vi "Vision Auto Move Straight.vi"(6 "Target Angle":dbl, 7 "Target Distance":dbl=15.0 format="%#_13g", 8 "Error In":errorcluster, 11 "Refnum's In":T1) -> (0 "Error Out":errorcluster, 3 "Refnum's Out":T1)   [LabVIEW 2018]
uses:
  <vilib>/Rock Robotics/WPI/ThirdParty/Phoenix-LabVIEW/Controls/CTRE_Phoenix_Params.ctl
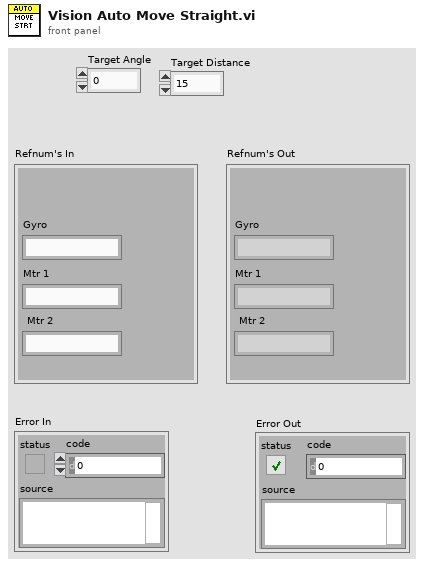
[diagram p1: front panel]
types:
  T1 = cluster{"Gyro":string, "Mtr 1":string, "Mtr 2":string}
  T2 = typedef "WPI_MotorControlDeviceRef.ctl" = cluster{"DeviceStatus":errorcluster, "Type":T3, "PWM":cluster{"PWM Channel":T4, "DeadBand":T5}, "CAN":cluster{"Device Number":u8, "SetOutput VI Ref":variant, "GetOutput VI Ref":variant, "Enable VI Ref":variant, "Disable VI Ref":variant, "Data":variant}, "Invert":bool, "DIO PWM":cluster{"PWM \"Enable\" Channel":T4, "DIOChannel":T6, "PWM Rate":dbl}}
  T3 = typedef "WPI_MotorControlType.ctl" = enum16{"PWM", "CAN", "DIO PWM"}
  T4 = typedef "FPGA_DIOPWMChannel.ctl" = enum8{"PWM 0", "PWM 1", "PWM 2", "PWM 3", "PWM 4", "PWM 5", "PWM 6", "PWM 7", "PWM 8", "PWM 9", "PWM MXP 0", "PWM MXP 1", "PWM MXP 2", "PWM MXP 3", "PWM MXP 4", "PWM MXP 5", "PWM MXP 6", "PWM MXP 7", "PWM MXP 8", "PWM MXP 9", "Invalid"}
  T5 = typedef "WPI_PWMDeadband.ctl" = cluster{"Name":string, "maxPositivePwm":i32, "minPositivePwm":i32, "centerPwm":i32, "maxNegativePwm":i32, "minNegativePwm":i32, "angularRange":u16}
  T6 = typedef "FPGA_DIOChannel.ctl" = enum8{"DIO 0", "DIO 1", "DIO 2", "DIO 3", "DIO 4", "DIO 5", "DIO 6", "DIO 7", "DIO 8", "DIO 9", "DIO MXP 0", "DIO MXP 1", "DIO MXP 2", "DIO MXP 3", "DIO MXP 4", "DIO MXP 5", "DIO MXP 6", "DIO MXP 7", "DIO MXP 8", "DIO MXP 9", "DIO MXP 10", "DIO MXP 11", "DIO MXP 12", "DIO MXP 13", "DIO MXP 14", "DIO MXP 15", "SPI Port CS1", "SPI Port CS2", "SPI Port CS3", "SPI Port MISO", "SPI Port MOSI", "Invalid"}
  T7 = typedef "WPI_GyroDevRef.ctl" = cluster{"DevStatus":errorcluster, "Analog Channel":T8, "Gain (VoltsPerDegree/Second)":dbl, "Gyro Type":enum16{"Analog", "XRS450"}, "Handle":i32, "SPI Bus":T9, "Device Found":bool, "Sample Rate":dbl, "Calibrate On Open":bool, "Offset":dbl}
  T8 = typedef "FPGA_AIChannel.ctl" = enum8{"AI 0", "AI 1", "AI 2", "AI 3", "AI MXP 0", "AI MXP 1", "AI MXP 2", "AI MXP 3", "Invalid"}
  T9 = typedef "spi_bus.ctl" = enum16{"SPI On-Board, CS0", "SPI On-Board, CS1", "SPI On-Board, CS2", "SPI On-Board, CS3", "SPI MXP", "Invalid"}
  T10 = typedef "CTRE_Phoenix_Params.ctl" = u16
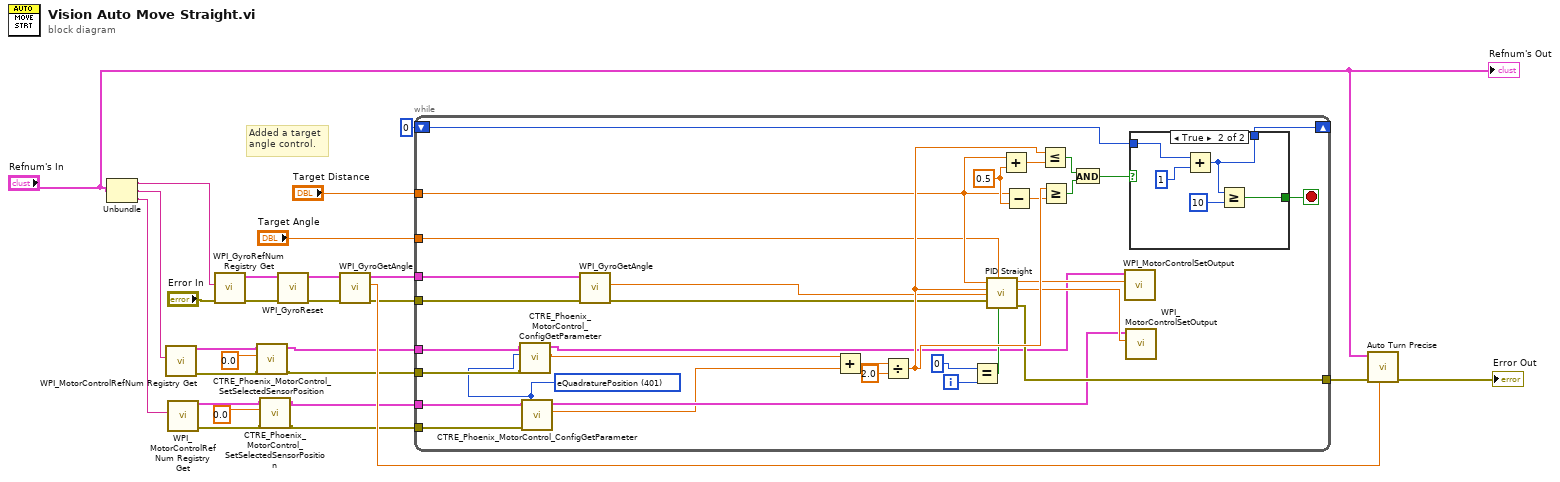
[diagram p0: block diagram]
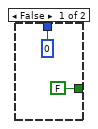
[diagram p2: hidden frame]
diagram:
  # "Added a target\nangle control."
  n1 = Unbundle("Refnum's In") -> ("Gyro"=w13:string, "Mtr 1"=w12:string, "Mtr 2"=w11:string)
  n2 = call <vilib>:"WPI_MotorControlRefNum Registry Get.vi"("refnum name"=w12) -> ("error out"=w4:errorcluster, "MotorControlDevRef"=w5:T2)  [unwired: 9 in]
  n3 = call <vilib>:"WPI_MotorControlRefNum Registry Get.vi"("refnum name"=w11) -> ("error out"=w7:errorcluster, "MotorControlDevRef"=w10:T2)  [unwired: 9 in]
  n4 = call <vilib>:"WPI_GyroRefNum Registry Get.vi"("error in (no error)"="Error In", "refnum name"=w13) -> ("error out"=w18:errorcluster, "GyroDevRef"=w17:T7)  [unwired: 8 in]
  n5 = call <vilib>:"CTRE_Phoenix_MotorControl_SetSelectedSensorPosition.vi"("error in (no error)"=w4, "New Sensor Position"=0.0, "PhoenixMotorControlDevRef"=w5) -> ("error out"=w3:errorcluster, "PhoenixMotorControlDevRef"=w2:T2)  [unwired: 7 in]
  n6 = call <vilib>:"CTRE_Phoenix_MotorControl_SetSelectedSensorPosition.vi"("error in (no error)"=w7, "New Sensor Position"=0.0, "PhoenixMotorControlDevRef"=w10) -> ("error out"=w8:errorcluster, "PhoenixMotorControlDevRef"=w9:T2)  [unwired: 7 in]
  n7 = call <vilib>:"WPI_GyroReset.vi"("error in"=w18, "GyroDevRef"=w17) -> ("error out"=w16:errorcluster, "GyroDevRef"=w15:T7)  [unwired: 8 in]
  n8 = call <vilib>:"WPI_GyroGetAngle.vi"("error in"=w16, "GyroDevRef"=w15) -> ("error out"=w20:errorcluster, "Angle"=w21:dbl, "GyroDevRef"=w19:T7)  [unwired: 5 in, 2 out]
  n9 = while {
    shift-right: [w49] -> _
    shift-left: 0 -> [w48]
    tunnel: "Target Distance" -> [w38]
    tunnel: [w44] -> w26
    tunnel: "Target Angle" -> [w37]
    tunnel: w19 -> [w40]
    tunnel: w20 -> [w39]
    tunnel: w8 -> [w35]
    tunnel: w9 -> [w36]
    tunnel: w3 -> [w32]
    tunnel: w2 -> [w33]
    i -> [w60]
    stop <- w43 stop-if-true
    w28 = T10 401 items=["eOnBoot_BrakeMode"=31, "eQuadFilterEn"=91, "eQuadIdxPolarity"=108, "eClearPositionOnIdx"=100, "eMotionProfileHasUnderrunErr"=119, "eMotionProfileTrajectoryPointDurationMs"=120, "eClearPosOnLimitF"=144, "eClearPosOnLimitR"=145, "eStatusFramePeriod"=300, "eOpenLoopRamp"=301, "eClosedLoopRamp"=302, "eNeutralDeadband"=303, "ePeakPosOutput"=305, "eNominalPosOutput"=306, "ePeakNegOutput"=307, "eNominalNegOutput"=308, "eProfileParamSlot_P"=310, "eProfileParamSlot_I"=311, "eProfileParamSlot_D"=312, "eProfileParamSlot_F"=313, "eProfileParamSlot_IZone"=314, "eProfileParamSlot_AllowableErr"=315, "eProfileParamSlot_MaxIAccum"=316, "eProfileParamSlot_PeakOutput"=317, "eClearPositionOnLimitF"=320, "eClearPositionOnLimitR"=321, "eClearPositionOnQuadIdx"=322, "eSampleVelocityPeriod"=325, "eSampleVelocityWindow"=326, "eFeedbackSensorType"=330, "eSelectedSensorPosition"=331, "eFeedbackNotContinuous"=332, "eRemoteSensorSource"=333, "eRemoteSensorDeviceID"=334, "eSensorTerm"=335, "eRemoteSensorClosedLoopDisableNeutralOnLOS"=336, "ePIDLoopPolarity"=337, "ePIDLoopPeriod"=338, "eSelectedSensorCoefficient"=339, "eForwardSoftLimitThreshold"=340, "eReverseSoftLimitThreshold"=341, "eForwardSoftLimitEnable"=342, "eReverseSoftLimitEnable"=343, "eNominalBatteryVoltage"=350, "eBatterVoltageFilterSize"=351, "eContinuousCurrentLimitAmps"=360, "eContinuousCurrentLimitMs"=361, "ePeakCurrentLimitAmps"=362, "eClosedLoopIAccum"=370, "eCustomParam"=380, "eStickyFaults"=390, "eAnalogPosition"=400, "eQuadraturePosition"=401, "ePulseWidthPosition"=402, "eMotMag_Accel"=410, "eMotMag_VelCruise"=411, "eLimitSwitchSource"=421, "eLimitSwitchNormClosedAndDis"=422, "eLimitSwitchDisabledNeutralOnLOS"=423, "eLimitSwitchRemoteDevID"=424, "eSoftLimitDisabledNeutralOnLOS"=425, "ePulseWidthPeriod_EdgesPerRot"=430, "ePulseWidthPeriod_FilterWindowSz"=431] ("Parameter")
    w56 = 0.5 ("y")
    n10 = call <vilib>:"CTRE_Phoenix_MotorControl_ConfigGetParameter.vi"("error in (no error)"=w32, "Parameter"=w28, "PhoenixMotorControlDevRef"=w33) -> ("value"=w30:dbl, "PhoenixMotorControlDevRef"=w31:T2)  [unwired: 6 in, 1 out]
    n11 = call <vilib>:"CTRE_Phoenix_MotorControl_ConfigGetParameter.vi"("error in (no error)"=w35, "Parameter"=w28, "PhoenixMotorControlDevRef"=w36) -> ("value"=w29:dbl, "PhoenixMotorControlDevRef"=w34:T2)  [unwired: 6 in, 1 out]
    n12 = call <vilib>:"WPI_GyroGetAngle.vi"("error in"=w39, "GyroDevRef"=w40) -> ("error out"=w45:errorcluster, "Angle"=w47:dbl)  [unwired: 5 in, 3 out]
    n13 = Add(x=w30, y=w29) -> (x+y=w57:dbl)
    n14 = Divide(x=w57, y=2.0) -> (x/y=w54:dbl)
    n15 = Equal?(x=0, y=w60) -> (x = y?=w46:bool)
    n16 = call "PID Straight.vi"("Reinitialize"=w46, "Target Angle"=w37, "Error In"=w45, "Gyro Angle"=w47, "Current Distance"=w54, "Target Distance"=w38) -> ("Error Out"=w44:errorcluster, "Right Power"=w41:dbl, "Left Power"=w42:dbl)  [unwired: 3 in]
    n17 = Add(x=w38, y=w56) -> (x+y=w55:dbl)
    n18 = Subtract(x=w38, y=w56) -> (x-y=w53:dbl)
    n19 = Less Or Equal?(x=w54, y=w55) -> (x <= y?=w52:bool)
    n20 = Greater Or Equal?(x=w54, y=w53) -> (x >= y?=w51:bool)
    n21 = And(x=w52, y=w51) -> (x .and. y?=w50:bool)
    n22 = call <vilib>:"WPI_MotorControlSetOutput.vi"("Output"=w42, "MotorControlDevRef"=w31) -> ()  [unwired: 7 in, 3 out]
    n23 = call <vilib>:"WPI_MotorControlSetOutput.vi"("Output"=w41, "MotorControlDevRef"=w34) -> ()  [unwired: 7 in, 3 out]
    n24 = case shown="True" w50 {
      tunnel: w48 -> [_ w66]
      tunnel: [0 w65] -> w49
      tunnel: [FALSE w63] -> w43
      frame False {
      }
      frame True {
        n25 = Add(x=w66, y=1) -> (x+y=w65:i32)
        n26 = Greater Or Equal?(x=w65, y=10) -> (x >= y?=w63:bool)
      }
    }
  }
  n27 = call "Auto Turn Precise.vi"("Target Distance"=w21, "Error In"=w26, "Refnum's In"="Refnum's In") -> ("Error Out"=→"Error Out":errorcluster)  [unwired: 7 in, 1 out]
  "Refnum's Out" <- "Refnum's In"
